vi "HRM-AQN-Simulated_read.vi"(8 "error in (no error)":errorcluster, 11 "AQN cluster in":T1) -> (0 "error out":errorcluster, 2 "data":waveform(dbl), 3 "AQN cluster out":T1)   [LabVIEW 2020]
uses:
  HRM-AQN-input_clust.ctl
  <vilib>/measure/NI_MABase.lvlib
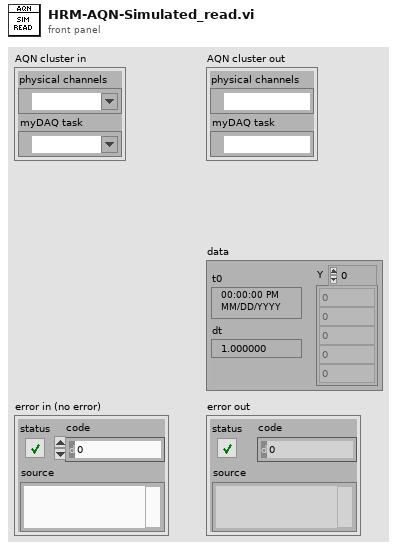
[diagram p1: front panel]
types:
  T1 = typedef "HRM-AQN-input_clust.ctl" = cluster{"physical channels":tag, "myDAQ task":refnum<k21>}
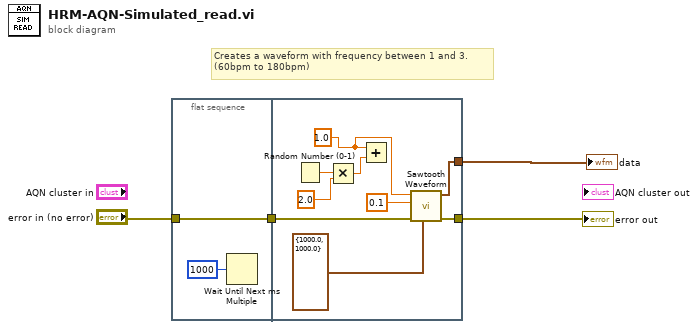
[diagram p0: block diagram]
diagram:
  # "Creates a waveform with frequency between 1 and 3.\n(60bpm to 180bpm)"
  n1 = flat-sequence {
    tunnel: "error in (no error)" -> [w6]
    tunnel: [w6] -> w2
    tunnel: [w14] -> w3
    tunnel: w2 -> [w15]
    tunnel: [w8] -> w1
    frame #0 {
      n2 = Wait Until Next ms Multiple(millisecond multiple=u32 1000) -> ()  [unwired: 1 out]
    }
    frame #1 {
      w7 = 1.0 ("frequency")
      n3 = Random Number (0-1)() -> (number: 0 to 1=w11:dbl)
      n4 = Multiply(x=w11, y=2.0) -> (x*y=w9:dbl)
      n5 = Add(x=w7, y=w9) -> ()  [unwired: 1 out]
      n6 = call <vilib>:"Sawtooth Waveform.vi"("sampling info"=cluster{"Fs":dbl, "#s":dbl} {"Fs"=1000.0, "#s"=1000.0}, "error in (no error)"=w15, "amplitude"=0.1, "frequency"=w7) -> ("error out"=w14:errorcluster, "signal out"=w8:waveform(dbl))  [unwired: 6 in]
    }
  }
  "data" <- w1
  "error out" <- w3
